vi "create with new queue.vi"(8 "error in":errorcluster) -> (0 "error out":errorcluster, 3 "identifying queue reporter out":refnum<class "identifying queue reporter.lvclass">)   [LabVIEW 2015, in "identifying queue reporter.lvclass"]
uses:
  identifying queue reporter.lvclass
  identifying queue reporter.lvclass/identifying queue reporter.ctl
  communicator queue/identifying queue.lvclass
panel:
  in  "size (1,10000)":i32=1000
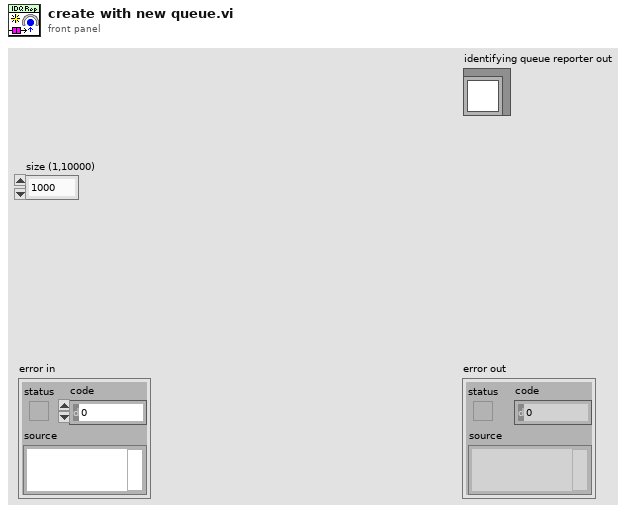
[diagram p1: front panel]
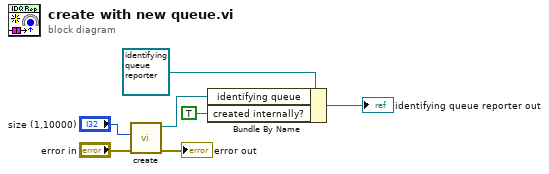
[diagram p0: block diagram]
diagram:
  n1 = call "create.vi"("error in"="error in", "size (1,10000)"="size (1,10000)") -> ("error out"=→"error out":errorcluster, "message connection out"=w1:refnum<class "identifying queue.lvclass">)  [unwired: 8 in]
  n2 = Bundle By Name(cluster=refnum<class "identifying queue reporter.lvclass"> refnum ("identifying queue reporter in"), "identifying queue"=w1, "created internally?"=TRUE) -> (→"identifying queue reporter out":refnum<class "identifying queue reporter.lvclass">)
